vi "ASG Add Delay.vi"(4 "Tailor Empty End (TRUE)":bool=TRUE, 6 "Tailor Empty Start (TRUE)":bool=TRUE, 7 "Round Time (to 1ns Precision)(TRUE)":bool=TRUE, 8 "error in":errorcluster, 10 "Channel delays(s)":dbl[](array[numeric]) format="%#_6p", 11 "Input Sequence":T3(xcontrol)=[{"Flags"=[TRUE, FALSE, FALSE, FALSE, FALSE, FALSE, FALSE, FALSE, FALSE, FALSE, FALSE, FALSE, FALSE, FALSE], "Comments"="", "Time"=2e-06, "Loop Config"={"Loop Code"=enum."Continued", "Number of Loop"=0, "End of Loop"=nan, "Loop Info"=""}}, {"Flags"=[TRUE, FALSE, TRUE, FALSE, FALSE, FALSE, FALSE, FALSE, FALSE, FALSE, FALSE, FALSE, FALSE, FALSE], "Comments"="", "Time"=5e-08, "Loop Config"={"Loop Code"=enum."Continued", "Number of Loop"=0, "End of Loop"=nan, "Loop Info"=""}}, {"Flags"=[TRUE, TRUE, FALSE, FALSE, FALSE, FALSE, FALSE, FALSE, FALSE, FALSE, FALSE, FALSE, FALSE, FALSE], "Comments"="", "Time"=5e-05, "Loop Config"={"Loop Code"=enum."Continued", "Number of Loop"=0, "End of Loop"=nan, "Loop Info"=""}}, {"Flags"=[TRUE, FALSE, TRUE, FALSE, FALSE, FALSE, FALSE, FALSE, FALSE, FALSE, FALSE, FALSE, FALSE, FALSE], "Comments"="", "Time"=5e-08, "Loop Config"={"Loop Code"=enum."Continued", "Number of Loop"=0, "End of Loop"=nan, "Loop Info"=""}}, {"Flags"=[TRUE, FALSE, FALSE, FALSE, FALSE, FALSE, FALSE, FALSE, TRUE, FALSE, FALSE, FALSE, FALSE, FALSE], "Comments"="", "Time"=2e-06, "Loop Config"={"Loop Code"=enum."Continued", "Number of Loop"=0, "End of Loop"=nan, "Loop Info"=""}}, {"Flags"=[TRUE, FALSE, TRUE, FALSE, FALSE, FALSE, FALSE, FALSE, FALSE, FALSE, FALSE, FALSE, FALSE, FALSE], "Comments"="", "Time"=5e-08, "Loop Config"={"Loop Code"=enum."Continued", "Number of Loop"=0, "End of Loop"=nan, "Loop Info"=""}}, {"Flags"=[TRUE, FALSE, FALSE, FALSE, FALSE, FALSE, FALSE, FALSE, FALSE, FALSE, FALSE, FALSE, FALSE, FALSE], "Comments"="", "Time"=5e-05, "Loop Config"={"Loop Code"=enum."Continued", "Number of Loop"=0, "End of Loop"=nan, "Loop Info"=""}}, {"Flags"=[TRUE, FALSE, TRUE, FALSE, FALSE, FALSE, FALSE, FALSE, FALSE, FALSE, FALSE, FALSE, FALSE, FALSE], "Comments"="", "Time"=5e-08, "Loop Config"={"Loop Code"=enum."Continued", "Number of Loop"=0, "End of Loop"=nan, "Loop Info"=""}}, {"Flags"=[TRUE, FALSE, FALSE, FALSE, FALSE, FALSE, FALSE, FALSE, FALSE, FALSE, FALSE, FALSE, FALSE, FALSE], "Comments"="", "Time"=2e-06, "Loop Config"={"Loop Code"=enum."Continued", "Number of Loop"=0, "End of Loop"=nan, "Loop Info"=""}}]) -> (0 "error out":errorcluster, 3 "Output Sequence":T3(xcontrol)=[{"Flags"=[TRUE, FALSE, FALSE, FALSE, FALSE, FALSE, FALSE, FALSE, FALSE, FALSE, FALSE, FALSE, FALSE, FALSE], "Comments"="", "Time"=2e-06, "Loop Config"={"Loop Code"=enum."Continued", "Number of Loop"=0, "End of Loop"=nan, "Loop Info"=""}}, {"Flags"=[TRUE, FALSE, TRUE, FALSE, FALSE, FALSE, FALSE, FALSE, FALSE, FALSE, FALSE, FALSE, FALSE, FALSE], "Comments"="", "Time"=5e-08, "Loop Config"={"Loop Code"=enum."Continued", "Number of Loop"=0, "End of Loop"=nan, "Loop Info"=""}}, {"Flags"=[TRUE, TRUE, FALSE, FALSE, FALSE, FALSE, FALSE, FALSE, FALSE, FALSE, FALSE, FALSE, FALSE, FALSE], "Comments"="", "Time"=5e-05, "Loop Config"={"Loop Code"=enum."Continued", "Number of Loop"=0, "End of Loop"=nan, "Loop Info"=""}}, {"Flags"=[TRUE, FALSE, TRUE, FALSE, FALSE, FALSE, FALSE, FALSE, FALSE, FALSE, FALSE, FALSE, FALSE, FALSE], "Comments"="", "Time"=5e-08, "Loop Config"={"Loop Code"=enum."Continued", "Number of Loop"=0, "End of Loop"=nan, "Loop Info"=""}}, {"Flags"=[TRUE, FALSE, FALSE, FALSE, FALSE, FALSE, FALSE, FALSE, TRUE, FALSE, FALSE, FALSE, FALSE, FALSE], "Comments"="", "Time"=2e-06, "Loop Config"={"Loop Code"=enum."Continued", "Number of Loop"=0, "End of Loop"=nan, "Loop Info"=""}}, {"Flags"=[TRUE, FALSE, TRUE, FALSE, FALSE, FALSE, FALSE, FALSE, FALSE, FALSE, FALSE, FALSE, FALSE, FALSE], "Comments"="", "Time"=5e-08, "Loop Config"={"Loop Code"=enum."Continued", "Number of Loop"=0, "End of Loop"=nan, "Loop Info"=""}}, {"Flags"=[TRUE, FALSE, FALSE, FALSE, FALSE, FALSE, FALSE, FALSE, FALSE, FALSE, FALSE, FALSE, FALSE, FALSE], "Comments"="", "Time"=5e-05, "Loop Config"={"Loop Code"=enum."Continued", "Number of Loop"=0, "End of Loop"=nan, "Loop Info"=""}}, {"Flags"=[TRUE, FALSE, TRUE, FALSE, FALSE, FALSE, FALSE, FALSE, FALSE, FALSE, FALSE, FALSE, FALSE, FALSE], "Comments"="", "Time"=5e-08, "Loop Config"={"Loop Code"=enum."Continued", "Number of Loop"=0, "End of Loop"=nan, "Loop Info"=""}}, {"Flags"=[TRUE, FALSE, FALSE, FALSE, FALSE, FALSE, FALSE, FALSE, FALSE, FALSE, FALSE, FALSE, FALSE, FALSE], "Comments"="", "Time"=2e-06, "Loop Config"={"Loop Code"=enum."Continued", "Number of Loop"=0, "End of Loop"=nan, "Loop Info"=""}}])   [LabVIEW 2020]
uses:
  Labview Library/Libraries/HW_LMMR_ASG8100/LMMR ASG/ASG Instructions XControl.xctl
panel:
  out "Sequence After Delay":T3(xcontrol)=[{"Flags"=[FALSE, TRUE, FALSE, FALSE, FALSE, FALSE, FALSE, FALSE, FALSE, FALSE, FALSE, FALSE, FALSE, FALSE], "Comments"="1/2pi", "Time"=-1.0, "Loop Config"={"Loop Code"=enum."Continued", "Number of Loop"=0, "End of Loop"=nan, "Loop Info"=""}}, {"Flags"=[FALSE, FALSE, FALSE, FALSE, FALSE, FALSE, FALSE, FALSE, FALSE, FALSE, FALSE, FALSE, FALSE, FALSE], "Comments"="tau", "Time"=-1.0, "Loop Config"={"Loop Code"=enum."Continued", "Number of Loop"=0, "End of Loop"=nan, "Loop Info"=""}}, {"Flags"=[FALSE, TRUE, FALSE, FALSE, FALSE, FALSE, FALSE, FALSE, FALSE, FALSE, FALSE, FALSE, FALSE, FALSE], "Comments"="1/2pi", "Time"=-1.0, "Loop Config"={"Loop Code"=enum."Continued", "Number of Loop"=0, "End of Loop"=nan, "Loop Info"=""}}, {"Flags"=[FALSE, FALSE, FALSE, FALSE, FALSE, FALSE, FALSE, FALSE, FALSE, FALSE, FALSE, FALSE, FALSE, FALSE], "Comments"="ReadSeq", "Time"=-1.0, "Loop Config"={"Loop Code"=enum."Continued", "Number of Loop"=0, "End of Loop"=nan, "Loop Info"=""}}, {"Flags"=[FALSE, TRUE, FALSE, FALSE, FALSE, FALSE, FALSE, FALSE, FALSE, FALSE, FALSE, FALSE, FALSE, FALSE], "Comments"="1/2pi", "Time"=-1.0, "Loop Config"={"Loop Code"=enum."Continued", "Number of Loop"=0, "End of Loop"=nan, "Loop Info"=""}}, {"Flags"=[FALSE, FALSE, FALSE, FALSE, FALSE, FALSE, FALSE, FALSE, FALSE, FALSE, FALSE, FALSE, FALSE, FALSE], "Comments"="tau", "Time"=-1.0, "Loop Config"={"Loop Code"=enum."Continued", "Number of Loop"=0, "End of Loop"=nan, "Loop Info"=""}}, {"Flags"=[FALSE, TRUE, FALSE, FALSE, FALSE, FALSE, FALSE, FALSE, FALSE, FALSE, FALSE, FALSE, FALSE, FALSE], "Comments"="3/2pi", "Time"=-1.0, "Loop Config"={"Loop Code"=enum."Continued", "Number of Loop"=0, "End of Loop"=nan, "Loop Info"=""}}, {"Flags"=[FALSE, FALSE, FALSE, FALSE, FALSE, FALSE, FALSE, FALSE, FALSE, FALSE, FALSE, FALSE, FALSE, FALSE], "Comments"="ReadSeq", "Time"=-1.0, "Loop Config"={"Loop Code"=enum."Continued", "Number of Loop"=0, "End of Loop"=nan, "Loop Info"=""}}]
  out "Time Sequence x 8 Channel With Delay":dbl[][](array[numeric]) format="%#_6p"
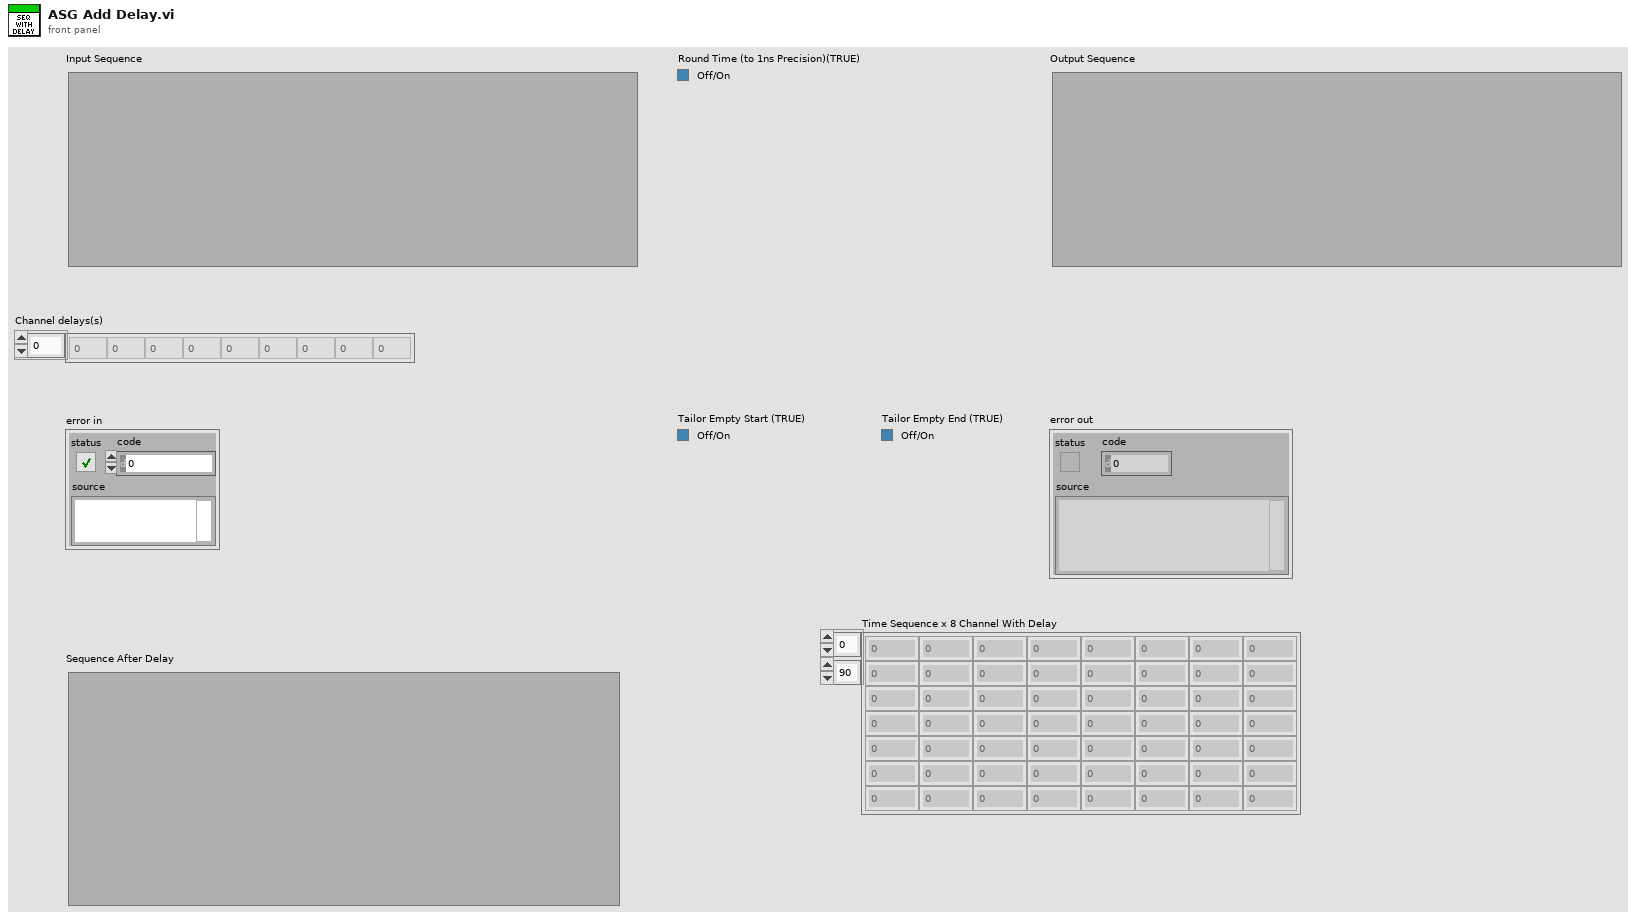
[diagram p1: front panel]
types:
  T1 = typedef "Loop XControl.xctl/Loop Config.ctl" = cluster{"Loop Code":T2, "Number of Loop":i32, "End of Loop":dbl, "Loop Info":string}
  T2 = typedef "Loop XControl.xctl/Loop Code.ctl" = enum16{"Continued", "Loop", "End Loop"}
  T3 = cluster{"Flags":bool[], "Comments":string, "Time":dbl, "Loop Config":T1}[]
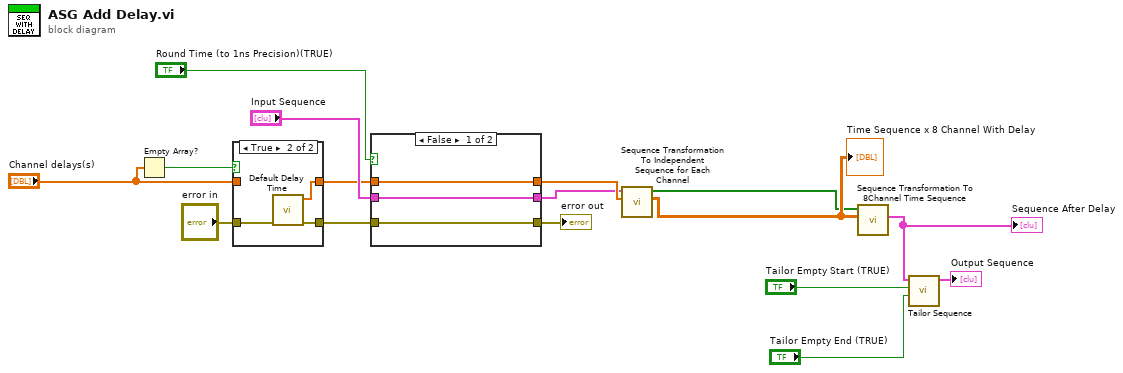
[diagram p0: block diagram]
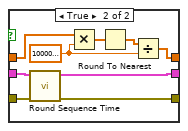
[diagram p3: hidden frame]
diagram:
  n1 = Empty Array?(array="Channel delays(s)") -> (empty?=w8:bool)
  n2 = case shown="True" w8 {
    tunnel: [w18 w21] -> w7
    tunnel: "Channel delays(s)" -> [w18 _]
    tunnel: "error in" -> [w17 w20]
    tunnel: [w17 w19] -> w4
    frame False {
    }
    frame True {
      n3 = call "Default Delay Time.vi"("error in (no error)"=w20) -> ("error out"=w19:errorcluster, "Delay Time"=w21:dbl[])  [unwired: 9 in]
    }
  }
  n4 = case shown="False" "Round Time (to 1ns Precision)(TRUE)" {
    tunnel: w7 -> [w23 w31]
    tunnel: [w23 w29] -> w13
    tunnel: w4 -> [w22 w28]
    tunnel: "Input Sequence" -> [w24 w27]
    tunnel: [w22 w26] -> w11
    tunnel: [w24 w25] -> w10
    frame False {
    }
    frame True {
      w30 = 1000000000.0 ("Numeric")
      n5 = call "Round Sequence Time.vi"("error in"=w28, "Input Sequence"=w27) -> ("error out"=w26:errorcluster, "Sequence After Round"=w25:T3)  [unwired: 8 in]
      n6 = Multiply(x=w31, y=w30) -> (x*y=w33:dbl[])
      n7 = Round To Nearest(number=w33) -> (nearest integer value=w32:dbl[])
      n8 = Divide(x=w32, y=w30) -> (x/y=w29:dbl[])
    }
  }
  "error out" <- w11
  n9 = call "Sequence Transformation To Independent Sequence for Each Channel.vi"("Channel delays(s)"=w13, "Array in"=w10) -> ("Time Sequence x 8 Channel"=w16:dbl[][], "Start Level x 8 Channel"=w15:bool[])  [unwired: 8 in]
  "Time Sequence x 8 Channel With Delay" <- w16
  n10 = call "Sequence Transformation To 8Channel Time Sequence.vi"("Time Sequence x 8 Channel"=w16, "Start Level x 8 Channel"=w15) -> ("8Channel Sequence"=w1:T3)  [unwired: 9 in]
  "Sequence After Delay" <- w1
  n11 = call "Tailor Sequence.vi"("Tailor Empty End (TRUE)"="Tailor Empty End (TRUE)", "Tailor Empty Start (TRUE)"="Tailor Empty Start (TRUE)", "8Channel Sequence in"=w1) -> ("8Channel Sequence out"=→"Output Sequence":T3)  [unwired: 8 in]
